vi "DriverVI.vi"() -> ()   [LabVIEW 2015]
panel:
  in  "Tab":enum32{"Com", "Digital", "Analog"}(tab)
  in  "DisconnectYldrm":bool
  in  "ConnectYldrm":bool
  in  "YLDRMPortInp":refnum<visa-resource-name>
  out "YLDRMErrorOut":errorcluster
  in  "Read 8 Dig Val":bool
  in  "Read Val":bool
  out "Read D Val":u8 max=1
  in  "PinDR":u8
  in  "Set Val":bool
  in  "Val":u8 max=1
  in  "PinDV":u8
  in  "Set Dir":bool
  in  "Dir":u8 max=1
  in  "PinDD":u8
  out "Digital Pin Array":bool[](array[boolean])
  in  "Read Real Time":bool
  out "VoltageB":dbl
  out "Voltage":dbl
  in  "PinAVB":u8=12 min=12 max=19
  in  "ReadAVB":u16 max=1
  in  "Read_AVB":bool
  in  "PinAV":u8=12 min=12 max=19
  in  "ReadAV":u16 max=1
  in  "Read_AV":bool
  out "AnValArr":dbl[](array[numeric]) format="%#.3g"
  # "kiesrd.com"
  # "0 to 7"
  # "kiesrd.com"
  # "kiesrd.com"
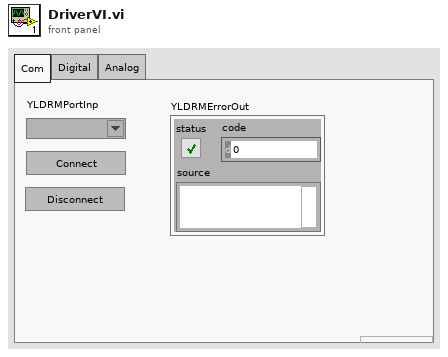
[diagram p1: front panel]
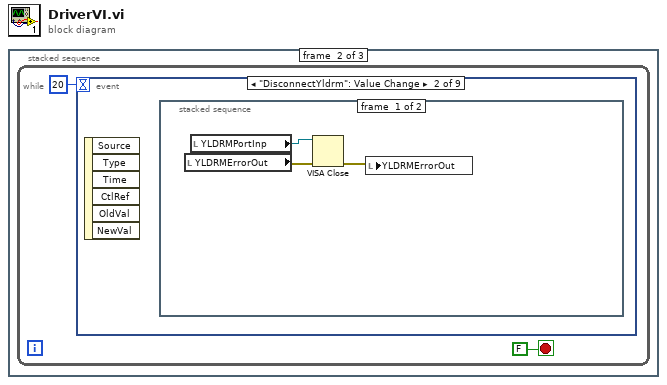
[diagram p0: block diagram]
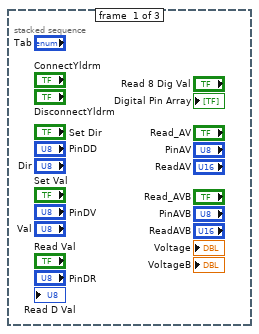
[diagram p2: hidden frame]
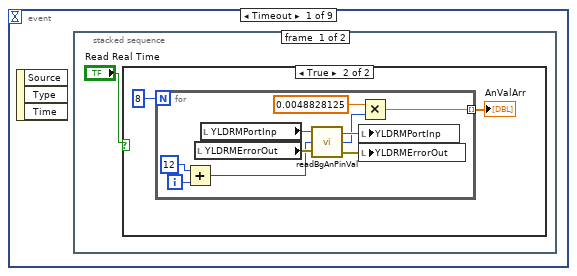
[diagram p3: hidden frame]
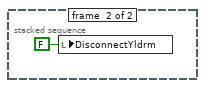
[diagram p6: hidden frame]
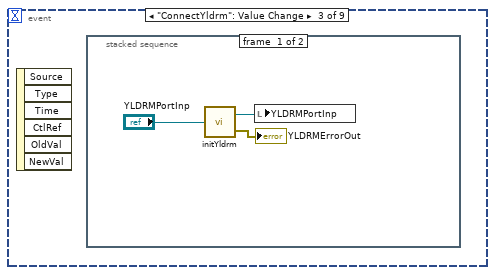
[diagram p7: hidden frame]
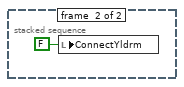
[diagram p8: hidden frame]
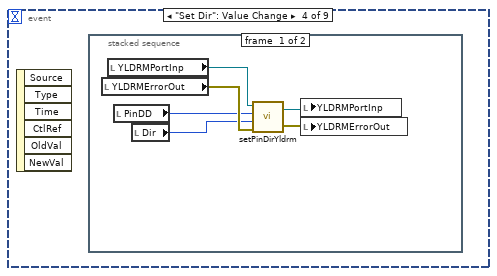
[diagram p9: hidden frame]
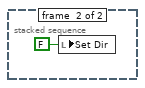
[diagram p10: hidden frame]
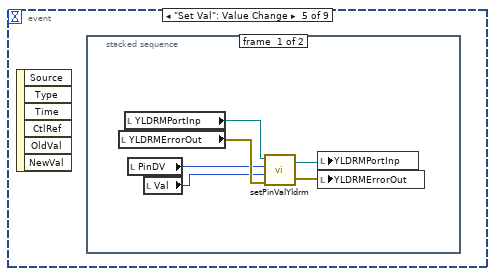
[diagram p11: hidden frame]
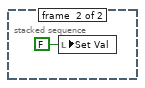
[diagram p12: hidden frame]
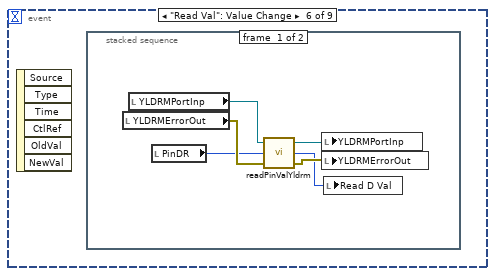
[diagram p13: hidden frame]
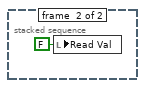
[diagram p14: hidden frame]
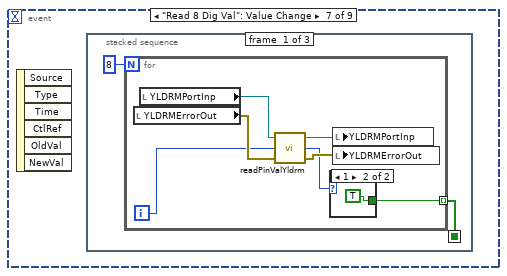
[diagram p15: hidden frame]
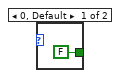
[diagram p16: hidden frame]
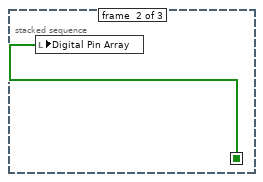
[diagram p17: hidden frame]
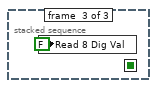
[diagram p18: hidden frame]
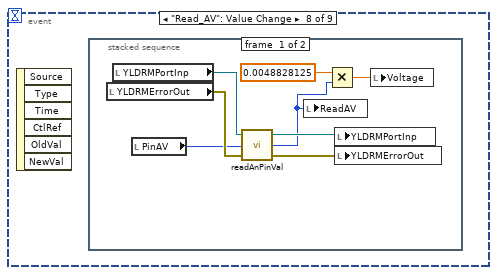
[diagram p19: hidden frame]
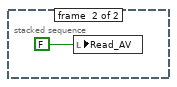
[diagram p20: hidden frame]
diagram:
  n1 = stacked-sequence {
    frame #0 {
    }
    frame #1 {
      n2 = while {
        stop <- FALSE stop-if-true
        n3 = event shown="[1] \"DisconnectYldrm\": Value Change" {
          selector: _ -> [_ _ _ _ _ _ _ _ _]
          dyn-events: _ -> [_ _ _ _ _ _ _ _ _]
          timeout: 20 -> [_ _ _ _ _ _ _ _ _]
          event Timeout {
            n4 = event-data() -> ()  [unwired: 1 in, 3 out]
            n5 = stacked-sequence {
              frame #0 {
                n6 = case shown="True" "Read Real Time" {
                  frame False {
                  }
                  frame True {
                    n7 = for {
                      N: 8 -> [_]
                      tunnel: [w6] -> w4 mode=indexing
                      i -> [w15]
                      n8 = Add(x=12, y=w15) -> (x+y=w7:i32)
                      n9 = local read "YLDRMErrorOut"() -> (w10:errorcluster)
                      n10 = local read "YLDRMPortInp"() -> (w11:refnum<visa-resource-name>)
                      n11 = call "readBgAnPinVal.vi"("YLDRMErrorInp"=w10, "pin"=w7, "YLDRMPortInp"=w11) -> ("YLDRMErrorOut"=w13:errorcluster, "out"=w9:u16, "YLDRMPortOut"=w12:refnum<visa-resource-name>)
                      n12 = local write "YLDRMPortInp"(w12) -> ()
                      n13 = local write "YLDRMErrorOut"(w13) -> ()
                      n14 = Multiply(x=0.0048828125, y=w9) -> (x*y=w6:dbl)
                    }
                    "AnValArr" <- w4
                  }
                }
              }
              frame #1 {
              }
            }
          }
          event "DisconnectYldrm": Value Change {
            n15 = event-data() -> ()  [unwired: 1 in, 6 out]
            n16 = stacked-sequence {
              frame #0 {
                n17 = local read "YLDRMErrorOut"() -> (w18:errorcluster)
                n18 = local read "YLDRMPortInp"() -> (w17:refnum<visa-resource-name>)
                n19 = VISA Close(VISA resource name=w17, error in (no error)=w18) -> (error out=w16:errorcluster)
                n20 = local write "YLDRMErrorOut"(w16) -> ()
              }
              frame #1 {
                n21 = local write "DisconnectYldrm"(FALSE ("DisconnectYldrm")) -> ()
              }
            }
          }
          event "ConnectYldrm": Value Change {
            n22 = event-data() -> ()  [unwired: 1 in, 6 out]
            n23 = stacked-sequence {
              frame #0 {
                n24 = call "initYldrm.vi"("YLDRMPortInp"="YLDRMPortInp") -> ("YLDRMPortOut"=w21:refnum<visa-resource-name>, "YLDRMErrorOut"=→"YLDRMErrorOut":errorcluster)
                n25 = local write "YLDRMPortInp"(w21) -> ()
              }
              frame #1 {
                n26 = local write "ConnectYldrm"(FALSE ("ConnectYldrm")) -> ()
              }
            }
          }
          event "Set Dir": Value Change {
            n27 = event-data() -> ()  [unwired: 1 in, 6 out]
            n28 = stacked-sequence {
              frame #0 {
                n29 = local read "YLDRMErrorOut"() -> (w28:errorcluster)
                n30 = local read "YLDRMPortInp"() -> (w29:refnum<visa-resource-name>)
                n31 = local read "PinDD"() -> (w27:u8)
                n32 = local read "Dir"() -> (w26:u8)
                n33 = call "setPinDirYldrm.vi"("YLDRMErrorInp"=w28, "dir"=w26, "pin"=w27, "YLDRMPortInp"=w29) -> ("YLDRMErrorOut"=w25:errorcluster, "YLDRMPortOut"=w24:refnum<visa-resource-name>)
                n34 = local write "YLDRMPortInp"(w24) -> ()
                n35 = local write "YLDRMErrorOut"(w25) -> ()
              }
              frame #1 {
                n36 = local write "Set Dir"(FALSE ("Set Dir")) -> ()
              }
            }
          }
          event "Set Val": Value Change {
            n37 = event-data() -> ()  [unwired: 1 in, 6 out]
            n38 = stacked-sequence {
              frame #0 {
                n39 = local read "YLDRMErrorOut"() -> (w33:errorcluster)
                n40 = local read "YLDRMPortInp"() -> (w34:refnum<visa-resource-name>)
                n41 = local read "PinDV"() -> (w32:u8)
                n42 = local read "Val"() -> (w31:u8)
                n43 = call "setPinValYldrm.vi"("YLDRMErrorInp"=w33, "val"=w31, "pin"=w32, "YLDRMPortInp"=w34) -> ("YLDRMErrorOut"=w36:errorcluster, "YLDRMPortOut"=w35:refnum<visa-resource-name>)
                n44 = local write "YLDRMPortInp"(w35) -> ()
                n45 = local write "YLDRMErrorOut"(w36) -> ()
              }
              frame #1 {
                n46 = local write "Set Val"(FALSE ("Set Dir")) -> ()
              }
            }
          }
          event "Read Val": Value Change {
            n47 = event-data() -> ()  [unwired: 1 in, 6 out]
            n48 = stacked-sequence {
              frame #0 {
                n49 = local read "YLDRMErrorOut"() -> (w40:errorcluster)
                n50 = local read "YLDRMPortInp"() -> (w41:refnum<visa-resource-name>)
                n51 = local read "PinDR"() -> (w39:u8)
                n52 = call "readPinValYldrm.vi"("YLDRMErrorInp"=w40, "pin"=w39, "YLDRMPortInp"=w41) -> ("YLDRMErrorOut"=w42:errorcluster, "out"=w38:u8, "YLDRMPortOut"=w43:refnum<visa-resource-name>)
                n53 = local write "YLDRMPortInp"(w43) -> ()
                n54 = local write "YLDRMErrorOut"(w42) -> ()
                n55 = local write "Read D Val"(w38) -> ()
              }
              frame #1 {
                n56 = local write "Read Val"(FALSE ("Set Dir")) -> ()
              }
            }
          }
          event "Read 8 Dig Val": Value Change {
            n57 = event-data() -> ()  [unwired: 1 in, 6 out]
            n58 = stacked-sequence {
              seq-local: [w45 _ _] -> [_ w56 _]
              frame #0 {
                n59 = for {
                  N: 8 -> [_]
                  tunnel: [w47] -> w45 mode=indexing
                  i -> [w49]
                  n60 = local read "YLDRMErrorOut"() -> (w50:errorcluster)
                  n61 = local read "YLDRMPortInp"() -> (w51:refnum<visa-resource-name>)
                  n62 = call "readPinValYldrm.vi"("YLDRMErrorInp"=w50, "pin"=w49, "YLDRMPortInp"=w51) -> ("YLDRMErrorOut"=w52:errorcluster, "out"=w48:u8, "YLDRMPortOut"=w53:refnum<visa-resource-name>)
                  n63 = case shown="1" w48 {
                    tunnel: [FALSE TRUE] -> w47
                    frame 0, Default {
                    }
                    frame 1 {
                    }
                  }
                  n64 = local write "YLDRMPortInp"(w53) -> ()
                  n65 = local write "YLDRMErrorOut"(w52) -> ()
                }
              }
              frame #1 {
                n66 = local write "Digital Pin Array"(w56) -> ()
              }
              frame #2 {
                n67 = local write "Read 8 Dig Val"(FALSE ("Set Dir")) -> ()
              }
            }
          }
          event "Read_AV": Value Change {
            n68 = event-data() -> ()  [unwired: 1 in, 6 out]
            n69 = stacked-sequence {
              frame #0 {
                n70 = local read "YLDRMErrorOut"() -> (w64:errorcluster)
                n71 = local read "YLDRMPortInp"() -> (w65:refnum<visa-resource-name>)
                n72 = local read "PinAV"() -> (w63:u8)
                n73 = call "readAnPinVal.vi"("YLDRMErrorInp"=w64, "pin"=w63, "YLDRMPortInp"=w65) -> ("YLDRMErrorOut"=w62:errorcluster, "out"=w58:u16, "YLDRMPortOut"=w61:refnum<visa-resource-name>)
                n74 = local write "ReadAV"(w58) -> ()
                n75 = Multiply(x=0.0048828125, y=w58) -> (x*y=w59:dbl)
                n76 = local write "YLDRMPortInp"(w61) -> ()
                n77 = local write "YLDRMErrorOut"(w62) -> ()
                n78 = local write "Voltage"(w59) -> ()
              }
              frame #1 {
                n79 = local write "Read_AV"(FALSE ("ConnectYldrm")) -> ()
              }
            }
          }
          event "Read_AVB": Value Change {
            n80 = event-data() -> ()  [unwired: 1 in, 6 out]
            n81 = stacked-sequence {
              frame #0 {
                n82 = local read "YLDRMErrorOut"() -> (w71:errorcluster)
                n83 = local read "YLDRMPortInp"() -> (w72:refnum<visa-resource-name>)
                n84 = local read "PinAVB"() -> (w70:u8)
                n85 = call "readBgAnPinVal.vi"("YLDRMErrorInp"=w71, "pin"=w70, "YLDRMPortInp"=w72) -> ("YLDRMErrorOut"=w74:errorcluster, "out"=w69:u16, "YLDRMPortOut"=w73:refnum<visa-resource-name>)
                n86 = Multiply(x=0.0048828125, y=w69) -> (x*y=w67:dbl)
                n87 = local write "ReadAVB"(w69) -> ()
                n88 = local write "YLDRMPortInp"(w73) -> ()
                n89 = local write "YLDRMErrorOut"(w74) -> ()
                n90 = local write "VoltageB"(w67) -> ()
              }
              frame #1 {
                n91 = local write "Read_AVB"(FALSE ("ConnectYldrm")) -> ()
              }
            }
          }
        }
      }
    }
    frame #2 {
      n92 = local read "YLDRMErrorOut"() -> (w77:errorcluster)
      n93 = local read "YLDRMPortInp"() -> (w78:refnum<visa-resource-name>)
      n94 = VISA Close(VISA resource name=w78, error in (no error)=w77) -> (error out=w76:errorcluster)
      n95 = local write "YLDRMErrorOut"(w76) -> ()
    }
  }
